vi "shooterReleaseControl.vi"(2 "Both":bool, 3 "shooterUpToSpeed":bool, 4 "Bottom":bool, 5 "Top":bool, 6 "Shotgun":bool, 7 "MachineGun":bool) -> (0 "bottomOpen":bool, 1 "topOpen":bool)   [LabVIEW 2012]
panel:
  in  "BeginShootDelay":dbl caption="Time Target (s)"
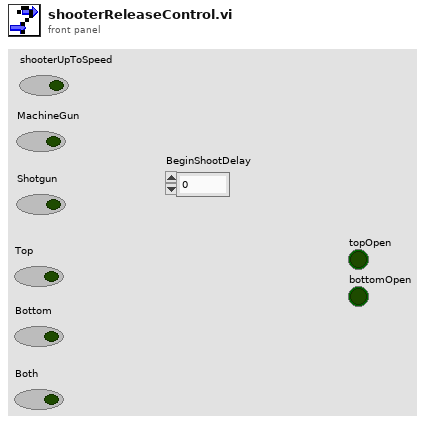
[diagram p1: front panel]
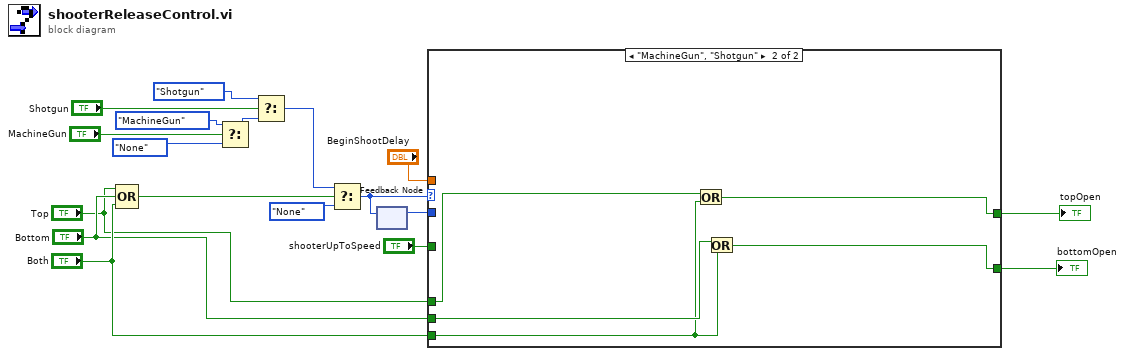
[diagram p0: block diagram]
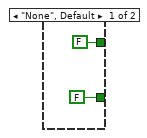
[diagram p2: hidden frame]
diagram:
  n1 = Compound Arithmetic op=OR("Top", "Bottom", "Both") -> (w10:bool)
  n2 = Select(t=enum16{"None", "MachineGun", "Shotgun"}."MachineGun", s="MachineGun", f=enum16{"None", "MachineGun", "Shotgun"}."None") -> (s? t:f=w18:enum16{"None", "MachineGun", "Shotgun"})
  n3 = Select(t=enum16{"None", "MachineGun", "Shotgun"}."Shotgun", s="Shotgun", f=w18) -> (s? t:f=w12:enum16{"None", "MachineGun", "Shotgun"})
  n4 = Select(t=w12, s=w10, f=enum16{"None", "MachineGun", "Shotgun"}."None") -> (s? t:f=w8:enum16{"None", "MachineGun", "Shotgun"})
  n5 = feedback #1() -> (w7:enum16{"None", "MachineGun", "Shotgun"})  [unwired: 1 in]
  n6 = feedback-in #1(w8) -> ()
  n7 = case shown="\"MachineGun\", \"Shotgun\"" w8 {
    tunnel: "shooterUpToSpeed" -> [_ _]
    tunnel: w7 -> [_ _]
    tunnel: "BeginShootDelay" -> [_ _]
    tunnel: [FALSE w22] -> w5
    tunnel: [FALSE w21] -> w4
    tunnel: "Both" -> [_ w23]
    tunnel: "Bottom" -> [_ w24]
    tunnel: "Top" -> [_ w25]
    frame "None", Default {
    }
    frame "MachineGun", "Shotgun" {
      n8 = Or(x=w25, y=w23) -> (x .or. y?=w22:bool)
      n9 = Or(x=w24, y=w23) -> (x .or. y?=w21:bool)
    }
  }
  "topOpen" <- w5
  "bottomOpen" <- w4
